vi "Keithley_2440_set_up.vi"() -> ()   [LabVIEW 2019]
uses:
  Equipment/Keithley 24XX/Keithley 24XX.lvlib
panel:
  out "Visa-Keithley-out":refnum<visa-resource-name>
  in  "Visa-Keithley-in":refnum<visa-resource-name>
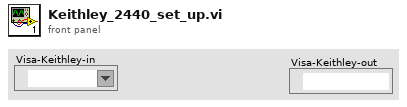
[diagram p1: front panel]
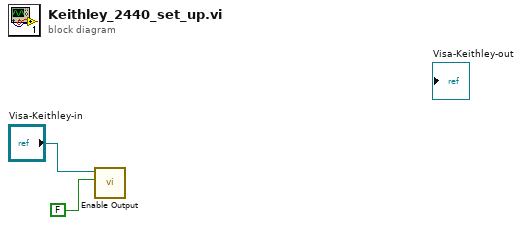
[diagram p0: block diagram]
diagram:
  n1 = call "Enable Output.vi"("Enable Output (T: Enable)"=FALSE, "VISA resource name"="Visa-Keithley-in") -> ()  [unwired: 8 in, 2 out]
